vi "DS3231_Decode_Temperature.vi"(7 "Data_Valid?":bool, 11 "DS3231.Temp_Data_In":u8[](array[numeric])) -> (3 "Temp.DegC_Out":dbl)   [LabVIEW 2022 SP3]
doc: "Petrus Prins\n31 July 2026"
uses:
  <vilib>/MakerHub/Toolbox/LMH-Toolbox.lvlib
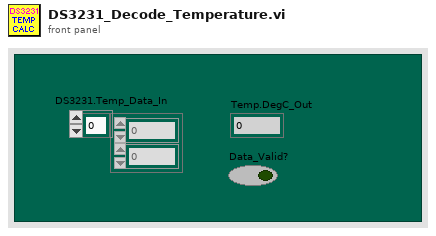
[diagram p1: front panel]
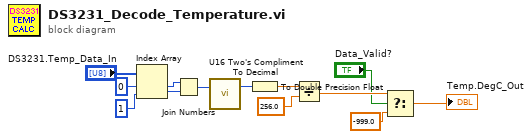
[diagram p0: block diagram]
diagram:
  n1 = Index Array(array="DS3231.Temp_Data_In", index #1=0 ("index"), index #2=1 ("index")) -> (element #1=w12:u8, element #2=w13:u8)
  n2 = Join Numbers(hi=w12, lo=w13) -> ((hi.lo)=w5:u16)
  n3 = call <vilib>:"U16 Two's Compliment To Decimal.vi"("Two's Compliment U16"=w5) -> ("Decimal I16"=w6:i16)  [unwired: 2 in]
  n4 = To Double Precision Float(number=w6) -> (double precision float=w7:dbl)
  n5 = Divide(x=w7, y=256.0) -> (x/y=w2:dbl)
  n6 = Select(t=w2, s="Data_Valid?", f=-999.0 ("t")) -> (s? t:f=→"Temp.DegC_Out":dbl)
